vi "Single Cursor Time Delta.vi"(8 "error in":errorcluster, 11 "Instrument Handle In":i32) -> (0 "error out":errorcluster, 2 "Delta Time":dbl, 3 "Instrument Handle Out":i32)   [LabVIEW 8.6, in "ZTScopeM.lvlib"]
doc: "Query the time difference between the cursor positions."
uses:
  ZTScopeM.lvlib
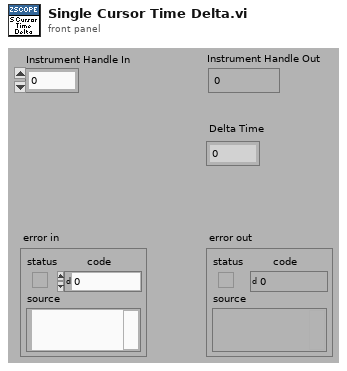
[diagram p1: front panel]
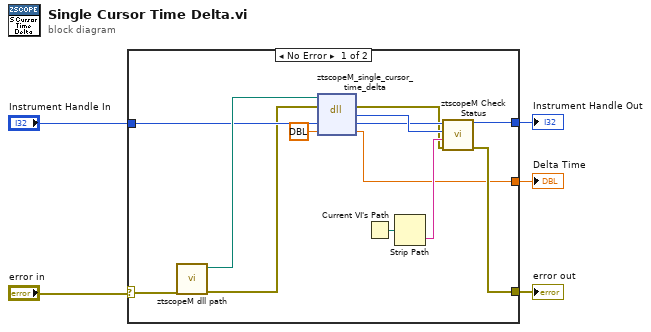
[diagram p0: block diagram]
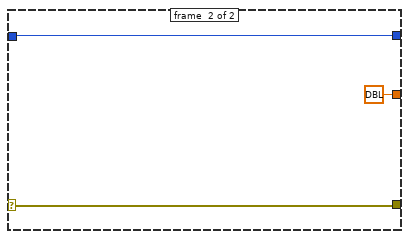
[diagram p2: hidden frame]
diagram:
  n1 = case shown="No Error" "error in" {
    selector: "error in" -> [w10 w21]
    tunnel: [w13 w21] -> w4
    tunnel: [w14 w19] -> w3
    tunnel: [w12 dbl ? ("cursorMagnitude")] -> w2
    tunnel: "Instrument Handle In" -> [w8 w19]
    frame #0 {
      n2 = call "ztscopeM dll path.vi"("error in (no error)"=w10) -> ("error out"=w7:errorcluster, "<instrument>.dll path"=w9:path)  [unwired: 9 in]
      n3 = dll-call lib="C:/Program Files (x86)/National Instruments/LabVIEW 2013/instr.lib/ztscopem/ztscopeM.dll" fn="ztscopeM_single_cursor_time_delta"(path in=w9, error in=w7, "instrumentHandle"=w8, "deltaTime"=dbl ?) -> (error out=w6:errorcluster, "return type"=w18:i32, "instrumentHandle"=w17:i32, "deltaTime"=w12:dbl)  [unwired: 1 in, 1 out]
      n4 = Current VI's Path() -> (path=w16:path)
      n5 = Strip Path(path=w16) -> (name=w15:string)  [unwired: 1 out]
      n6 = call "ztscopeM Check Status.vi"("error in"=w6, "name of VI"=w15, "status (return code)"=w18, "instrument handle in"=w17) -> ("error out"=w13:errorcluster, "instrument handle out"=w14:i32)  [unwired: 2 out]
    }
    frame #1 {
    }
  }
  "Instrument Handle Out" <- w3
  "error out" <- w4
  "Delta Time" <- w2
